vi "LOGIC_CreateWhen.vi"(11 "Database RefNum in":T1) -> (1 "onexpstart":bool, 2 "onreadend":bool, 3 "onreadstart":bool)   [LabVIEW 2016]
uses:
  DBSHAND/private/vis/DatabaseHand_RefNum.ctl
  DBSHAND/private/vis/DatabaseHand_Element_Get(string).vi
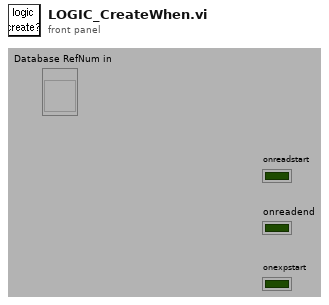
[diagram p1: front panel]
types:
  T1 = typedef "DatabaseHand_RefNum.ctl" = refnum<vi>
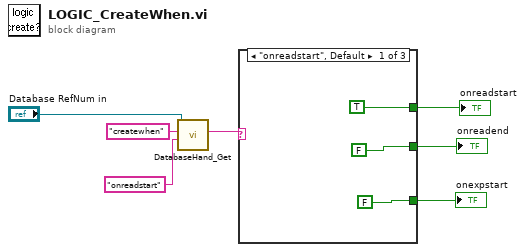
[diagram p0: block diagram]
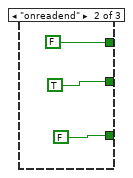
[diagram p2: hidden frame]
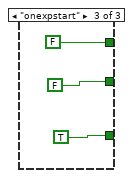
[diagram p3: hidden frame]
diagram:
  n1 = call-poly "DatabaseHand_Get.vi"("default value"="onreadstart", "name"="createwhen", "Database RefNum in"="Database RefNum in") -> ("value"=w4:string)  [unwired: 2 in, 6 out]
  n2 = case shown="\"onreadstart\", Default" w4 {
    tunnel: [TRUE FALSE FALSE] -> w3
    tunnel: [FALSE ("onreadend") TRUE ("onreadend") FALSE ("onreadend")] -> w2
    tunnel: [FALSE ("onreadend") FALSE ("onreadend") TRUE ("onreadend")] -> w1
    frame "onreadstart", Default {
    }
    frame "onreadend" {
    }
    frame "onexpstart" {
    }
  }
  "onreadstart" <- w3
  "onreadend" <- w2
  "onexpstart" <- w1
